vi "Get Variant Value.vi"(11 "Variant in":variant) -> (3 "Variant value as string":string)   [LabVIEW 2014]
doc: "Returns datatype as string from wired input. It tries to convert it to others datatypes and when it is possible it add this datatype into output list.\nSo if there is variant type i32 (32bit integer) it returns array ['double','i32'] because this value can be converted to double as well as to i32. solution is always take last array value."
uses:
  <vilib>/Utility/VariantDataType/Type.ctl
  <vilib>/Utility/VariantDataType/VariantType.lvlib
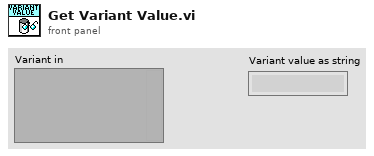
[diagram p1: front panel]
types:
  T1 = typedef "VariantType.lvlib/Type.ctl" = enum8{"Invalid Type", "Void", "I8", "I16", "I32", "I64", "U8", "U16", "U32", "U64", "Single Float", "Double Float", "Extended Float", "Single Complex", "Double Complex", "Extended Complex", "Enum U8", "Enum U16", "Enum U32", "Enum U64", "Single Float With Unit", "Double Float With Unit", "Extended Float With Unit", "Single Complex with Unit", "Double Complex with Unit", "Extended Complex with Unit", "Boolean", "String", "Path", "Picture", "Tag", "Array", "Cluster", "Variant", "LV Variant", "Waveform", "Timestamp", "Digital Waveform", "Digital Data", "ExpressData", "Refnum", "External Data", "VI", "Poly VI", "LabVIEW Class Instance", "Fixed Point"}
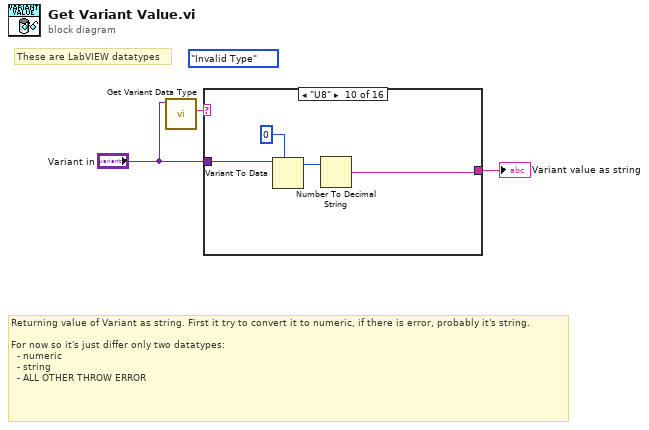
[diagram p0: block diagram]
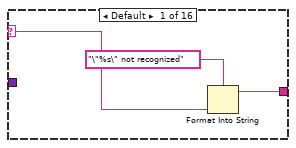
[diagram p2: hidden frame]
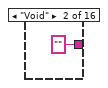
[diagram p3: hidden frame]
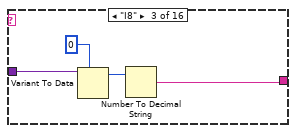
[diagram p4: hidden frame]
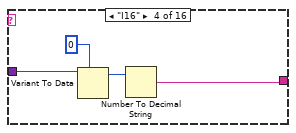
[diagram p5: hidden frame]
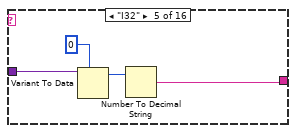
[diagram p6: hidden frame]
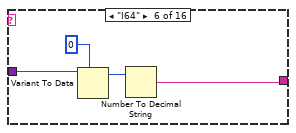
[diagram p7: hidden frame]
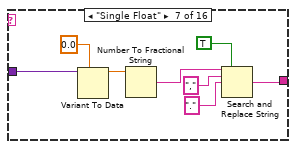
[diagram p8: hidden frame]
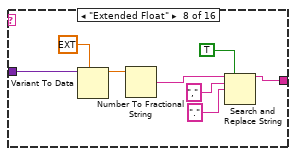
[diagram p9: hidden frame]
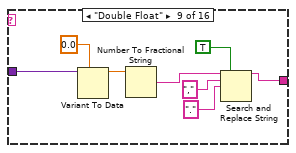
[diagram p10: hidden frame]
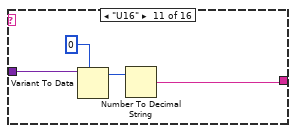
[diagram p11: hidden frame]
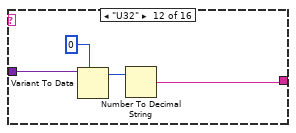
[diagram p12: hidden frame]
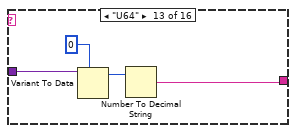
[diagram p13: hidden frame]
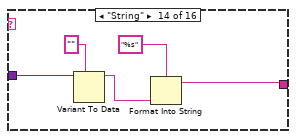
[diagram p14: hidden frame]
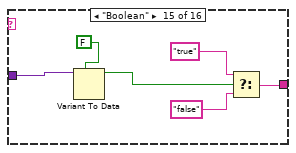
[diagram p15: hidden frame]
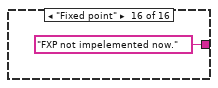
[diagram p16: hidden frame]
diagram:
  (unwired) Type."Invalid Type" ("LabVIEW Variant Data Types")
  # "These are LabVIEW datatypes"
  # "Returning value of Variant as string. First it try to convert it to numeric, if there is error, probably it's string.\n\nFor now so it's just differ only two datatypes:\n  - numeric\n  - string\n  - ALL OTHER THROW ERROR"
  n1 = call "Get Variant Data Type.vi"("Variant in"="Variant in") -> ("first data type"=w2:string)  [unwired: 9 in, 1 out]
  n2 = case shown="\"U8\"" w2 {
    selector: w2 -> [w5 _ _ _ _ _ _ _ _ _ _ _ _ _ _ _]
    tunnel: [w6 "" w9 w13 w17 w21 w28 w33 w41 w49 w53 w57 w61 w66 w71 "FXP not impelemented now."] -> w3
    tunnel: "Variant in" -> [_ _ w11 w15 w19 w23 w31 w39 w47 w51 w55 w59 w63 w68 w74 _]
    frame Default {
      n3 = Format Into String(format string="\"%s\" not recognized", w5) -> (resulting string=w6:string)  [unwired: 2 in, 1 out]
    }
    frame "Void" {
    }
    frame "I8" {
      n4 = Variant To Data(type=i8 0, Variant=w11) -> (data=w8:i8)  [unwired: 1 in, 1 out]
      n5 = Number To Decimal String(number=w8) -> (decimal integer string=w9:string)  [unwired: 1 in]
    }
    frame "I16" {
      n6 = Variant To Data(type=i16 0, Variant=w15) -> (data=w12:i16)  [unwired: 1 in, 1 out]
      n7 = Number To Decimal String(number=w12) -> (decimal integer string=w13:string)  [unwired: 1 in]
    }
    frame "I32" {
      n8 = Variant To Data(type=0, Variant=w19) -> (data=w16:i32)  [unwired: 1 in, 1 out]
      n9 = Number To Decimal String(number=w16) -> (decimal integer string=w17:string)  [unwired: 1 in]
    }
    frame "I64" {
      n10 = Variant To Data(type=i64 0, Variant=w23) -> (data=w20:i64)  [unwired: 1 in, 1 out]
      n11 = Number To Decimal String(number=w20) -> (decimal integer string=w21:string)  [unwired: 1 in]
    }
    frame "Single Float" {
      n12 = Variant To Data(type=0.0, Variant=w31) -> (data=w29:dbl)  [unwired: 1 in, 1 out]
      n13 = Number To Fractional String(number=w29) -> (F-format string=w27:string)  [unwired: 3 in]
      n14 = Search and Replace String(replace all?=TRUE ("replace all? (F)"), input string=w27, search string=",", replace string="." ("search string")) -> (result string=w28:string)  [unwired: 4 in, 3 out]
    }
    frame "Extended Float" {
      n15 = Variant To Data(type=ext 0.0, Variant=w39) -> (data=w37:ext)  [unwired: 1 in, 1 out]
      n16 = Number To Fractional String(number=w37) -> (F-format string=w32:string)  [unwired: 3 in]
      n17 = Search and Replace String(replace all?=TRUE ("replace all? (F)"), input string=w32, search string=",", replace string="." ("search string")) -> (result string=w33:string)  [unwired: 4 in, 3 out]
    }
    frame "Double Float" {
      n18 = Variant To Data(type=sgl 0.0, Variant=w47) -> (data=w45:sgl)  [unwired: 1 in, 1 out]
      n19 = Number To Fractional String(number=w45) -> (F-format string=w40:string)  [unwired: 3 in]
      n20 = Search and Replace String(replace all?=TRUE ("replace all? (F)"), input string=w40, search string=",", replace string="." ("search string")) -> (result string=w41:string)  [unwired: 4 in, 3 out]
    }
    frame "U8" {
      n21 = Variant To Data(type=u8 0, Variant=w51) -> (data=w48:u8)  [unwired: 1 in, 1 out]
      n22 = Number To Decimal String(number=w48) -> (decimal integer string=w49:string)  [unwired: 1 in]
    }
    frame "U16" {
      n23 = Variant To Data(type=u16 0, Variant=w55) -> (data=w52:u16)  [unwired: 1 in, 1 out]
      n24 = Number To Decimal String(number=w52) -> (decimal integer string=w53:string)  [unwired: 1 in]
    }
    frame "U32" {
      n25 = Variant To Data(type=u32 0, Variant=w59) -> (data=w56:u32)  [unwired: 1 in, 1 out]
      n26 = Number To Decimal String(number=w56) -> (decimal integer string=w57:string)  [unwired: 1 in]
    }
    frame "U64" {
      n27 = Variant To Data(type=u64 0, Variant=w63) -> (data=w60:u64)  [unwired: 1 in, 1 out]
      n28 = Number To Decimal String(number=w60) -> (decimal integer string=w61:string)  [unwired: 1 in]
    }
    frame "String" {
      n29 = Variant To Data(type="", Variant=w68) -> (data=w65:string)  [unwired: 1 in, 1 out]
      n30 = Format Into String(format string="%s", w65) -> (resulting string=w66:string)  [unwired: 2 in, 1 out]
    }
    frame "Boolean" {
      n31 = Variant To Data(type=FALSE, Variant=w74) -> (data=w72:bool)  [unwired: 1 in, 1 out]
      n32 = Select(t="true", s=w72, f="false") -> (s? t:f=w71:string)
    }
    frame "Fixed point" {
    }
  }
  "Variant value as string" <- w3
